vi "Trial timings file.vi"(7 "Operations":enum16{"Create", "Write", "Close"}(ring), 8 "error in (no error)":errorcluster, 11 "Array":u64[](array[numeric])) -> (0 "error out":errorcluster)   [LabVIEW 2017]
uses:
  Global Variables/General Globals.vi
panel:
  out "timings":u64[](array[numeric])
  out "Array 3":u64[](array[numeric])
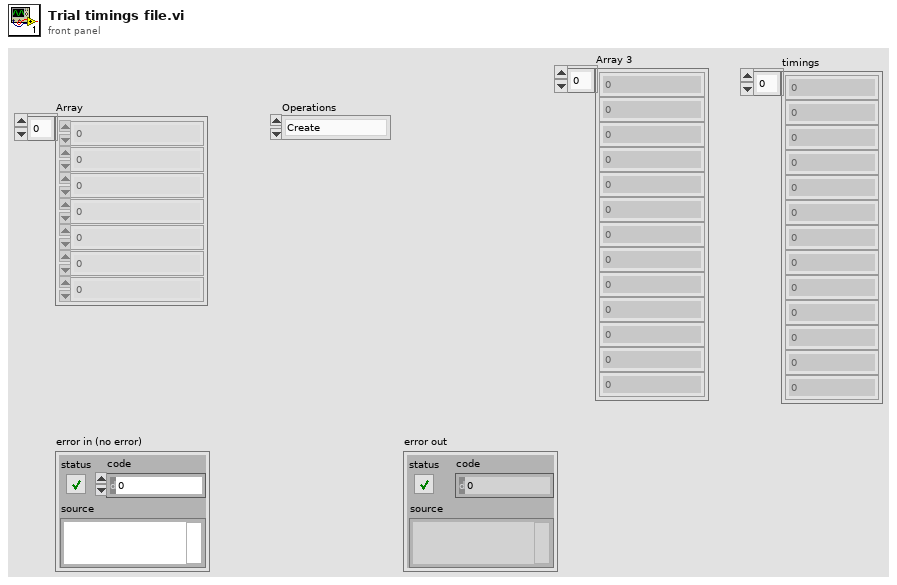
[diagram p1: front panel]
types:
  T1 = enum16{"open", "replace", "create", "open or create", "replace or create", "replace or create with confirmation"}
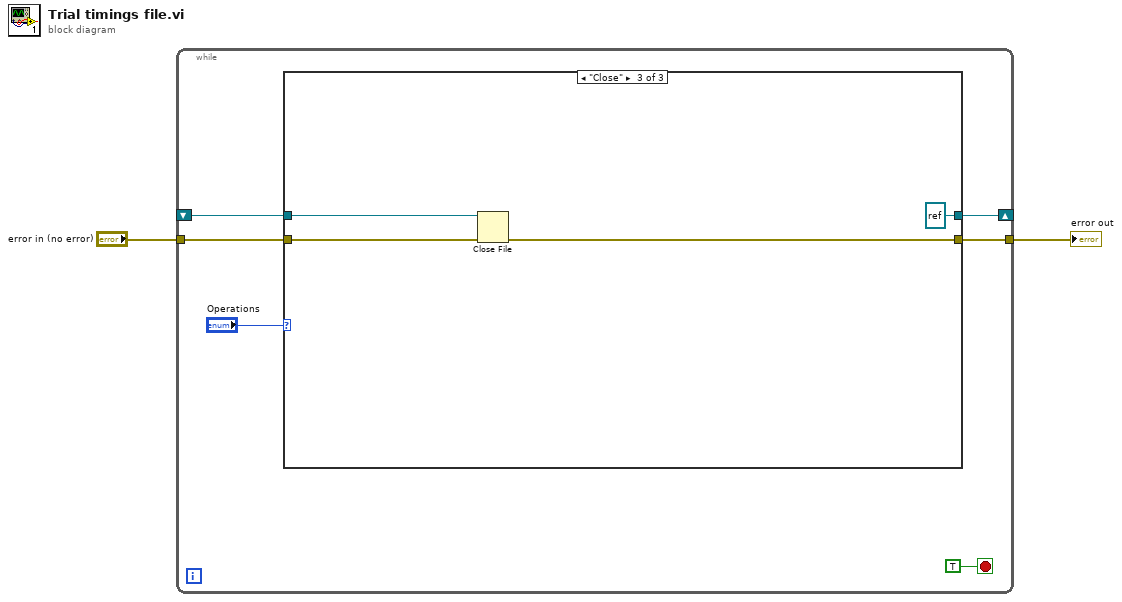
[diagram p0: block diagram]
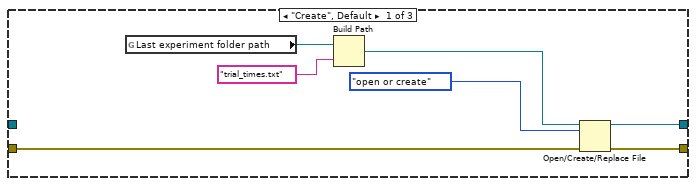
[diagram p2: hidden frame]
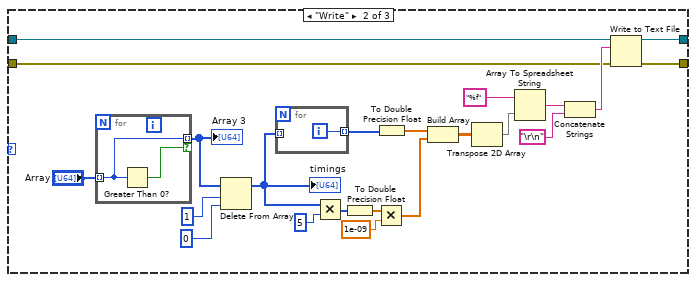
[diagram p3: hidden frame]
diagram:
  n1 = while {
    shift-right: [w6] -> _
    shift-left: _ -> [w5]
    tunnel: "error in (no error)" -> [w3]
    tunnel: [w4] -> w1
    stop <- TRUE stop-if-true
    n2 = case shown="\"Close\"" "Operations" {
      tunnel: [w11 w36 refnum<file> refnum ("refnum out")] -> w6
      tunnel: w5 -> [_ w37 w44]
      tunnel: [w10 w16 w42] -> w4
      tunnel: w3 -> [w9 w17 w43]
      frame "Create", Default {
        n3 = global read "General Globals.vi" "Last experiment folder path"() -> (w15:path)
        n4 = Build Path(base path=w15, name or relative path="trial_times.txt") -> (appended path=w13:path)
        n5 = Open/Create/Replace File(file path (use dialog)=w13, error in=w9, operation (0:open)=T1."open or create") -> (refnum out=w11:refnum<file>, error out=w10:errorcluster)  [unwired: 3 in, 1 out]
      }
      frame "Write" {
        n6 = for {
          tunnel: "Array" -> [w40] mode=indexing
          tunnel: [w40] -> w35 mode=indexing if=w39
          n7 = Greater Than 0?(x=w40) -> (x > 0?=w39:bool)
        }
        "Array 3" <- w35
        n8 = Delete From Array(array=w35, length=1, index=0) -> (array with subset deleted=w22:u64[])  [unwired: 1 out]
        "timings" <- w22
        n9 = for {
          tunnel: w22 -> [_] mode=indexing
          tunnel: [w38] -> w21 mode=indexing
          i -> [w38]
        }
        n10 = Multiply(x=w22, y=u64 5) -> (x*y=w30:u64[])
        n11 = To Double Precision Float(number=w30) -> (double precision float=w29:dbl[])
        n12 = Multiply(x=w29, y=1e-09) -> (x*y=w27:dbl[])
        n13 = To Double Precision Float(number=w21) -> (double precision float=w26:dbl[])
        n14 = Build Array(w26, w27) -> (w25:dbl[][])
        n15 = Transpose 2D Array(2D array=w25) -> (transposed array=w23:dbl[][])
        n16 = Array To Spreadsheet String(array=w23, 3:"%f" ("format string")) -> (spreadsheet string=w20:string)  [unwired: 1 in]
        n17 = Concatenate Strings(w20, "\r\n") -> (w18:string)
        n18 = Write to Text File(file (use dialog)=w37, text=w18, error in=w17) -> (refnum out=w36:refnum<file>, error out=w16:errorcluster)  [unwired: 1 in, 1 out]
      }
      frame "Close" {
        n19 = Close File(refnum=w44, error in=w43) -> (error out=w42:errorcluster)  [unwired: 1 out]
      }
    }
  }
  "error out" <- w1
